vi "Eye Movement Analyser.vi"(7 "Data Output":T12) -> ()   [LabVIEW 2016] (continued)
          shift-left: dbl[][] [] -> [w1559]
          n741 = Unbundle By Name(w1562) -> ("List 1"=w1561:u16)
          n742 = Unbundle By Name(w1564) -> ("Data Channels"=w1563:dbl[][])
          n743 = Index Array(array=w1563, index (row)=w1561) -> (element=w1560:dbl[])  [unwired: 1 in]
          n744 = Build Array (concatenate)(w1559, w1560) -> (w1558:dbl[][])
        }
        n745 = Unbundle By Name(w1512) -> ("Sample Rate"=w1528:i32)
        n746 = stacked-sequence {
          tunnel: [_ w1552 _ _] -> w1514
          tunnel: [_ _ _ w1554] -> w1513
          frame #0 {
            n747 = property on="Time series Trace" class="WFGraph (strict)"("Active Cursor"=u32 0) -> ()  [unwired: 2 in, 2 out]
          }
          frame #1 {
            n748 = property on="Time series Trace" class="WFGraph (strict)"() -> ("Cursor.Cursor Position:Cursor X"=w1552:dbl)  [unwired: 2 in, 2 out]
          }
          frame #2 {
            n749 = property on="Time series Trace" class="WFGraph (strict)"("Active Cursor"=u32 1) -> ()  [unwired: 2 in, 2 out]
          }
          frame #3 {
            n750 = property on="Time series Trace" class="WFGraph (strict)"() -> ("Cursor.Cursor Position:Cursor X"=w1554:dbl)  [unwired: 2 in, 2 out]
          }
        }
        n751 = Multiply(x=w1514, y=w1528) -> (x*y=w1543:dbl)
        n752 = Multiply(x=w1513, y=w1528) -> (x*y=w1544:dbl)
        n753 = Subtract(x=w1544, y=w1543) -> (x-y=w1542:dbl)
        n754 = Decrement(x=w1542) -> (x-1=w1541:dbl)
        n755 = Array Subset(array=w1545, index (col)=w1543, length (col)=w1542) -> (w1526:dbl[][])  [unwired: 2 in]
        n756 = call-poly <vilib>:"Ramp Pattern.vi"("start"=0.0, "end"=w1541, "samples"=w1542) -> ("Ramp Pattern"=w1539:dbl[])  [unwired: 7 in, 1 out]
        n757 = for {
          tunnel: w1526 -> [w1557] mode=indexing
          tunnel: w1539 -> [w1556]
          tunnel: [w1555] -> w1527 mode=indexing
          n758 = call <vilib>:"Linear Fit.vi"("Y"=w1557, "X"=w1556) -> ("Best Linear Fit"=w1555:dbl[])  [unwired: 9 in, 4 out]
        }
        n759 = call-poly <vilib>:"Unit Vector.vi"("Input Vector"=w1518) -> ("Unit Vector"=w1511:dbl[])  [unwired: 8 in, 2 out]
        n760 = call-poly <vilib>:"Unit Vector.vi"("Input Vector"=w1517) -> ("Unit Vector"=w1510:dbl[])  [unwired: 8 in, 2 out]
        n761 = call-poly <vilib>:"Unit Vector.vi"("Input Vector"=w1516) -> ("Unit Vector"=w1508:dbl[])  [unwired: 8 in, 2 out]
        n762 = call "RotationVector_to_Quaternion-2.vi"("rotation vectors"=w1527) -> ("quaternions"=w1535:dbl[][])  [unwired: 4 in]
        n763 = Build Array (concatenate)(w1526, w1527) -> (w1504:dbl[][])
        "Fits a line to a noisy slow-phase. First 3 channels in plot window (above) must be x, y, and z eye position in that order." <- w1504
        n764 = call "Differentiate 3D.vi"("Sample Rate 4"=w1528, "Data (in)"=w1535) -> ("Data (differentiated)"=w1529:dbl[][])  [unwired: 3 in]
        n765 = call "Inverse_Quaternion-2.vi"("quaternions"=w1535) -> ("inverse quaternions"=w1530:dbl[][])  [unwired: 4 in]
        n766 = Index Array(array=w1504) -> (element #1=w1503:dbl[], element #2=w1502:dbl[], element #3=w1499:dbl[])  [unwired: 6 in]
        n767 = call "QuaternionMultiplication.vi"("quaternions B"=w1530, "quaternions A"=w1529) -> ("quaternions A x B"=w1531:dbl[][])  [unwired: 3 in]
        n768 = Divide(x=360.0, y=3.141592653589793) -> (x/y=w1534:dbl)
        n769 = Multiply(x=w1531, y=w1534) -> (x*y=w1538:dbl[][])
        n770 = call "mean_nan.vi"("Array"=w1503) -> ("Mean"=→"Mean Ch 1":dbl)  [unwired: 10 in]
        n771 = call "mean_nan.vi"("Array"=w1502) -> ("Mean"=→"Mean Ch2":dbl)  [unwired: 10 in]
        n772 = call "mean_nan.vi"("Array"=w1499) -> ("Mean"=→"Mean Ch3":dbl)  [unwired: 10 in]
        n773 = Array Subset(array=w1538, index (row)=1 ("Array Index"), length (row)=3 ("Array Index")) -> (w1525:dbl[][])  [unwired: 2 in]
        n774 = Index Array(array=w1525, index (col)=1 ("index")) -> (element=w1524:dbl[])  [unwired: 1 in]
        "X deg/s      Y deg/s      Z deg/s" <- w1524
        n775 = call-poly <vilib>:"Unit Vector.vi"("Input Vector"=w1524) -> ("Unit Vector"=w1509:dbl[])  [unwired: 8 in, 2 out]
        n776 = call-poly <vilib>:"Dot Product.vi"("Y Vector"=w1511, "X Vector"=w1509) -> ("X * Y"=w1522:dbl)  [unwired: 1 out]
        n777 = call-poly <vilib>:"Dot Product.vi"("Y Vector"=w1510, "X Vector"=w1509) -> ("X * Y"=w1523:dbl)  [unwired: 1 out]
        n778 = call-poly <vilib>:"Dot Product.vi"("Y Vector"=w1508, "X Vector"=w1509) -> ("X * Y"=w1521:dbl)  [unwired: 1 out]
        n779 = Build Array(w1522, w1523, w1521) -> (w1520:dbl[])
        n780 = Absolute Value(x=w1520) -> (abs(x)=→"HOR\n\nLARP\n\nRALP":dbl[])
      }
      frame "Mars 3D" {
        n781 = Unbundle By Name(w1568) -> ("DC file"=w1569:path)
        n782 = call "Mars3D_new.vi"("Statemachine Data IN"=w1573, "File"=w1569) -> ("stop 3"=w1572:bool, "Statemachine Data OUT"=w1570:T30)  [unwired: 8 in]
        n783 = case shown="False" w1572 {
          tunnel: [w1584 w1586] -> w1571
          tunnel: w1570 -> [w1583 w1585]
          tunnel: [w1578 w1585] -> w1565
          frame False {
            w1584 = T14[] [enum."Make Batch List", enum."Generate New Time Plot", enum."Find default parameter"] items=["--- System ---", "Panel Monitoring", "Check Save Status", "Initialize", "Initialise GUI", "Quit", "--- Import ---", "Desaccade Time Data", "Desaccade Time Data Background", "Paint Delete", "Load Batch Log File", "Make Batch List", "Update Batch List", "Delete Batch List", "Delete Temporary LVS", "Save Temporary LVS", "Check for Batch LVS", "Process 3D Chinchilla", "Find default parameter", "Mars3D old", "Chair", "EyeSeeCam", "Open last session", "Save RAW", "Auto Impulse Parameter", "Save Image", "Wireless", "Process Coils Data", "Process JHOC Data", "Process Animal Data", "Australian Data", "ASCII", "Mars 3D", "Mars 3D Training", "Position Mean Plugin", "plot generator plugin", "Human VOG system", "Optotrak", "spline", "COR", "galvanic", "Generate New Time Plot", "Make off and gains permanent", "Generate New Impulse Plot", "Defer Impulse Plot", "Fill Impulse Plot Data", "Scale Impulse Plot", "Un-Defer Impulse Plot", "Snap Impulse Cursor", "Extract Saccades", "Impulse Analyser", "NTA", "Acceleration", "Saccade Velocity", "Horizontal Align", "Vertical Align", "Delete Impulse", "Cut Before", "Cut After", "Filter Data", "Undo Last", "Redo", "Mean and STD", "Group Analyser", "Generate Report", "Phase Plots", "Gain and Phase", "Example Plugin", "Time Constant Plugin", "Export Data", "Export Time Series Data", "Append Data", "Save Data", "Load Data", "Cut in Range", "Keep in range", "Stop"] ("State stack IN")
            w1582 = 1 ("index")
            # "Use Parameter Set 0"
            n784 = Bundle By Name(cluster=w1583, "Autosort Parameter Set"=w1582) -> (w1577:T30)
            n785 = property on="Autosize Parameter Set" class="Ring (strict)"("Val(Sgnl)"=w1582) -> ()  [unwired: 2 in, 2 out]
            n786 = property on="Impulse Trace" class="WFGraph (strict)"("Value"=cluster{dbl, dbl, "Impulses":dbl[][]} {0.0, 5.0, "Impulses"=[]} ("Impulse Trace")) -> ()  [unwired: 2 in, 2 out]
            n787 = Bundle By Name(cluster=w1577, "History Length"=0, "Histpry Position"=-1, "Undo Counter"=0) -> (w1578:T30)
            n788 = property on="Tab Control" class="TabCtl (strict)"("Value"=T1."Batch Process" ("Tab Control")) -> ()  [unwired: 2 in, 2 out]
          }
          frame True {
            w1586 = T14[] [enum."Panel Monitoring"] items=["--- System ---", "Panel Monitoring", "Check Save Status", "Initialize", "Initialise GUI", "Quit", "--- Import ---", "Desaccade Time Data", "Desaccade Time Data Background", "Paint Delete", "Load Batch Log File", "Make Batch List", "Update Batch List", "Delete Batch List", "Delete Temporary LVS", "Save Temporary LVS", "Check for Batch LVS", "Process 3D Chinchilla", "Find default parameter", "Mars3D old", "Chair", "EyeSeeCam", "Open last session", "Save RAW", "Auto Impulse Parameter", "Save Image", "Wireless", "Process Coils Data", "Process JHOC Data", "Process Animal Data", "Australian Data", "ASCII", "Mars 3D", "Mars 3D Training", "Position Mean Plugin", "plot generator plugin", "Human VOG system", "Optotrak", "spline", "COR", "galvanic", "Generate New Time Plot", "Make off and gains permanent", "Generate New Impulse Plot", "Defer Impulse Plot", "Fill Impulse Plot Data", "Scale Impulse Plot", "Un-Defer Impulse Plot", "Snap Impulse Cursor", "Extract Saccades", "Impulse Analyser", "NTA", "Acceleration", "Saccade Velocity", "Horizontal Align", "Vertical Align", "Delete Impulse", "Cut Before", "Cut After", "Filter Data", "Undo Last", "Redo", "Mean and STD", "Group Analyser", "Generate Report", "Phase Plots", "Gain and Phase", "Example Plugin", "Time Constant Plugin", "Export Data", "Export Time Series Data", "Append Data", "Save Data", "Load Data", "Cut in Range", "Keep in range", "Stop"] ("State stack IN")
            # "If operation was canceld"
          }
        }
        n789 = Bundle By Name(cluster=w1568, "DC file"=path "") -> (w1567:T17)
      }
      frame "Chair" {
        n790 = Unbundle By Name(w1594) -> ("DC file"=w1589:path)
        n791 = call "Chair Plugin.vi"("DC File"=w1589, "Data IN"=w1591) -> ("Cancelled"=w1588:bool, "Data OUT"=w1590:T30)  [unwired: 8 in]
        n792 = case shown="False" w1588 {
          tunnel: [w1606 w1608] -> w1595
          tunnel: w1590 -> [w1605 w1607]
          tunnel: [w1600 w1607] -> w1587
          frame False {
            w1606 = T14[] [enum."Make Batch List", enum."Generate New Time Plot", enum."Find default parameter"] items=["--- System ---", "Panel Monitoring", "Check Save Status", "Initialize", "Initialise GUI", "Quit", "--- Import ---", "Desaccade Time Data", "Desaccade Time Data Background", "Paint Delete", "Load Batch Log File", "Make Batch List", "Update Batch List", "Delete Batch List", "Delete Temporary LVS", "Save Temporary LVS", "Check for Batch LVS", "Process 3D Chinchilla", "Find default parameter", "Mars3D old", "Chair", "EyeSeeCam", "Open last session", "Save RAW", "Auto Impulse Parameter", "Save Image", "Wireless", "Process Coils Data", "Process JHOC Data", "Process Animal Data", "Australian Data", "ASCII", "Mars 3D", "Mars 3D Training", "Position Mean Plugin", "plot generator plugin", "Human VOG system", "Optotrak", "spline", "COR", "galvanic", "Generate New Time Plot", "Make off and gains permanent", "Generate New Impulse Plot", "Defer Impulse Plot", "Fill Impulse Plot Data", "Scale Impulse Plot", "Un-Defer Impulse Plot", "Snap Impulse Cursor", "Extract Saccades", "Impulse Analyser", "NTA", "Acceleration", "Saccade Velocity", "Horizontal Align", "Vertical Align", "Delete Impulse", "Cut Before", "Cut After", "Filter Data", "Undo Last", "Redo", "Mean and STD", "Group Analyser", "Generate Report", "Phase Plots", "Gain and Phase", "Example Plugin", "Time Constant Plugin", "Export Data", "Export Time Series Data", "Append Data", "Save Data", "Load Data", "Cut in Range", "Keep in range", "Stop"] ("State stack IN")
            w1604 = 10 ("index")
            # "Use Parameter Set"
            n793 = Bundle By Name(cluster=w1605, "Autosort Parameter Set"=w1604) -> (w1599:T30)
            n794 = property on="Autosize Parameter Set" class="Ring (strict)"("Val(Sgnl)"=w1604) -> ()  [unwired: 2 in, 2 out]
            n795 = property on="Impulse Trace" class="WFGraph (strict)"("Value"=cluster{dbl, dbl, "Impulses":dbl[][]} {0.0, 5.0, "Impulses"=[]} ("Impulse Trace")) -> ()  [unwired: 2 in, 2 out]
            n796 = Bundle By Name(cluster=w1599, "History Length"=0, "Histpry Position"=-1, "Undo Counter"=0) -> (w1600:T30)
            n797 = property on="Tab Control" class="TabCtl (strict)"("Value"=T1."Batch Process" ("Tab Control")) -> ()  [unwired: 2 in, 2 out]
          }
          frame True {
            w1608 = T14[] [enum."Panel Monitoring"] items=["--- System ---", "Panel Monitoring", "Check Save Status", "Initialize", "Initialise GUI", "Quit", "--- Import ---", "Desaccade Time Data", "Desaccade Time Data Background", "Paint Delete", "Load Batch Log File", "Make Batch List", "Update Batch List", "Delete Batch List", "Delete Temporary LVS", "Save Temporary LVS", "Check for Batch LVS", "Process 3D Chinchilla", "Find default parameter", "Mars3D old", "Chair", "EyeSeeCam", "Open last session", "Save RAW", "Auto Impulse Parameter", "Save Image", "Wireless", "Process Coils Data", "Process JHOC Data", "Process Animal Data", "Australian Data", "ASCII", "Mars 3D", "Mars 3D Training", "Position Mean Plugin", "plot generator plugin", "Human VOG system", "Optotrak", "spline", "COR", "galvanic", "Generate New Time Plot", "Make off and gains permanent", "Generate New Impulse Plot", "Defer Impulse Plot", "Fill Impulse Plot Data", "Scale Impulse Plot", "Un-Defer Impulse Plot", "Snap Impulse Cursor", "Extract Saccades", "Impulse Analyser", "NTA", "Acceleration", "Saccade Velocity", "Horizontal Align", "Vertical Align", "Delete Impulse", "Cut Before", "Cut After", "Filter Data", "Undo Last", "Redo", "Mean and STD", "Group Analyser", "Generate Report", "Phase Plots", "Gain and Phase", "Example Plugin", "Time Constant Plugin", "Export Data", "Export Time Series Data", "Append Data", "Save Data", "Load Data", "Cut in Range", "Keep in range", "Stop"] ("State stack IN")
            # "If operation was canceld"
          }
        }
        n798 = Bundle By Name(cluster=w1594, "DC file"=path "") -> (w1593:T17)
      }
      frame "EyeSeeCam" {
        n799 = Unbundle By Name(w1616) -> ("DC file"=w1609:path)
        n800 = call "EyeSeeCam Plugin.vi"("DC File"=w1609, "Data IN"=w1612) -> ("Cancelled"=w1610:bool, "Data OUT"=w1611:T30)  [unwired: 8 in]
        n801 = case shown="False" w1610 {
          tunnel: [w1628 w1630] -> w1617
          tunnel: w1611 -> [w1627 w1629]
          tunnel: [w1622 w1629] -> w1613
          frame False {
            w1628 = T14[] [enum."Make Batch List", enum."Generate New Time Plot", enum."Find default parameter"] items=["--- System ---", "Panel Monitoring", "Check Save Status", "Initialize", "Initialise GUI", "Quit", "--- Import ---", "Desaccade Time Data", "Desaccade Time Data Background", "Paint Delete", "Load Batch Log File", "Make Batch List", "Update Batch List", "Delete Batch List", "Delete Temporary LVS", "Save Temporary LVS", "Check for Batch LVS", "Process 3D Chinchilla", "Find default parameter", "Mars3D old", "Chair", "EyeSeeCam", "Open last session", "Save RAW", "Auto Impulse Parameter", "Save Image", "Wireless", "Process Coils Data", "Process JHOC Data", "Process Animal Data", "Australian Data", "ASCII", "Mars 3D", "Mars 3D Training", "Position Mean Plugin", "plot generator plugin", "Human VOG system", "Optotrak", "spline", "COR", "galvanic", "Generate New Time Plot", "Make off and gains permanent", "Generate New Impulse Plot", "Defer Impulse Plot", "Fill Impulse Plot Data", "Scale Impulse Plot", "Un-Defer Impulse Plot", "Snap Impulse Cursor", "Extract Saccades", "Impulse Analyser", "NTA", "Acceleration", "Saccade Velocity", "Horizontal Align", "Vertical Align", "Delete Impulse", "Cut Before", "Cut After", "Filter Data", "Undo Last", "Redo", "Mean and STD", "Group Analyser", "Generate Report", "Phase Plots", "Gain and Phase", "Example Plugin", "Time Constant Plugin", "Export Data", "Export Time Series Data", "Append Data", "Save Data", "Load Data", "Cut in Range", "Keep in range", "Stop"] ("State stack IN")
            w1626 = 10 ("index")
            # "Use Parameter Set"
            n802 = Bundle By Name(cluster=w1627, "Autosort Parameter Set"=w1626) -> (w1621:T30)
            n803 = property on="Autosize Parameter Set" class="Ring (strict)"("Val(Sgnl)"=w1626) -> ()  [unwired: 2 in, 2 out]
            n804 = property on="Impulse Trace" class="WFGraph (strict)"("Value"=cluster{dbl, dbl, "Impulses":dbl[][]} {0.0, 5.0, "Impulses"=[]} ("Impulse Trace")) -> ()  [unwired: 2 in, 2 out]
            n805 = Bundle By Name(cluster=w1621, "History Length"=0, "Histpry Position"=-1, "Undo Counter"=0) -> (w1622:T30)
            n806 = property on="Tab Control" class="TabCtl (strict)"("Value"=T1."Batch Process" ("Tab Control")) -> ()  [unwired: 2 in, 2 out]
          }
          frame True {
            w1630 = T14[] [enum."Panel Monitoring"] items=["--- System ---", "Panel Monitoring", "Check Save Status", "Initialize", "Initialise GUI", "Quit", "--- Import ---", "Desaccade Time Data", "Desaccade Time Data Background", "Paint Delete", "Load Batch Log File", "Make Batch List", "Update Batch List", "Delete Batch List", "Delete Temporary LVS", "Save Temporary LVS", "Check for Batch LVS", "Process 3D Chinchilla", "Find default parameter", "Mars3D old", "Chair", "EyeSeeCam", "Open last session", "Save RAW", "Auto Impulse Parameter", "Save Image", "Wireless", "Process Coils Data", "Process JHOC Data", "Process Animal Data", "Australian Data", "ASCII", "Mars 3D", "Mars 3D Training", "Position Mean Plugin", "plot generator plugin", "Human VOG system", "Optotrak", "spline", "COR", "galvanic", "Generate New Time Plot", "Make off and gains permanent", "Generate New Impulse Plot", "Defer Impulse Plot", "Fill Impulse Plot Data", "Scale Impulse Plot", "Un-Defer Impulse Plot", "Snap Impulse Cursor", "Extract Saccades", "Impulse Analyser", "NTA", "Acceleration", "Saccade Velocity", "Horizontal Align", "Vertical Align", "Delete Impulse", "Cut Before", "Cut After", "Filter Data", "Undo Last", "Redo", "Mean and STD", "Group Analyser", "Generate Report", "Phase Plots", "Gain and Phase", "Example Plugin", "Time Constant Plugin", "Export Data", "Export Time Series Data", "Append Data", "Save Data", "Load Data", "Cut in Range", "Keep in range", "Stop"] ("State stack IN")
            # "If operation was canceld"
          }
        }
        n807 = Bundle By Name(cluster=w1616, "DC file"=path "") -> (w1615:T17)
      }
      frame "Mars3D old" {
        n808 = call "Mars3D_old.vi"("Statemachine Data IN"=w1636) -> ("stop 3"=w1635:bool, "Statemachine Data OUT"=w1633:T30)  [unwired: 8 in, 1 out]
        n809 = case shown="False" w1635 {
          tunnel: [w1646 w1648] -> w1634
          tunnel: w1633 -> [w1644 w1647]
          tunnel: [w1638 w1647] -> w1631
          frame False {
            w1646 = T14[] [enum."Generate New Time Plot", enum."Find default parameter"] items=["--- System ---", "Panel Monitoring", "Check Save Status", "Initialize", "Initialise GUI", "Quit", "--- Import ---", "Desaccade Time Data", "Desaccade Time Data Background", "Paint Delete", "Load Batch Log File", "Make Batch List", "Update Batch List", "Delete Batch List", "Delete Temporary LVS", "Save Temporary LVS", "Check for Batch LVS", "Process 3D Chinchilla", "Find default parameter", "Mars3D old", "Chair", "EyeSeeCam", "Open last session", "Save RAW", "Auto Impulse Parameter", "Save Image", "Wireless", "Process Coils Data", "Process JHOC Data", "Process Animal Data", "Australian Data", "ASCII", "Mars 3D", "Mars 3D Training", "Position Mean Plugin", "plot generator plugin", "Human VOG system", "Optotrak", "spline", "COR", "galvanic", "Generate New Time Plot", "Make off and gains permanent", "Generate New Impulse Plot", "Defer Impulse Plot", "Fill Impulse Plot Data", "Scale Impulse Plot", "Un-Defer Impulse Plot", "Snap Impulse Cursor", "Extract Saccades", "Impulse Analyser", "NTA", "Acceleration", "Saccade Velocity", "Horizontal Align", "Vertical Align", "Delete Impulse", "Cut Before", "Cut After", "Filter Data", "Undo Last", "Redo", "Mean and STD", "Group Analyser", "Generate Report", "Phase Plots", "Gain and Phase", "Example Plugin", "Time Constant Plugin", "Export Data", "Export Time Series Data", "Append Data", "Save Data", "Load Data", "Cut in Range", "Keep in range", "Stop"] ("State stack IN")
            w1643 = 1 ("index")
            # "Use Parameter Set 0"
            n810 = Bundle By Name(cluster=w1644, "Autosort Parameter Set"=w1643) -> (w1639:T30)
            n811 = property on="Autosize Parameter Set" class="Ring (strict)"("Val(Sgnl)"=w1643) -> ()  [unwired: 2 in, 2 out]
            n812 = local write "Tab Control"(T1."Time series Parameter" ("Tab Control")) -> ()
            n813 = Bundle By Name(cluster=w1639, "History Length"=0, "Histpry Position"=-1, "Undo Counter"=0) -> (w1638:T30)
          }
          frame True {
            w1648 = T14[] [enum."Panel Monitoring"] items=["--- System ---", "Panel Monitoring", "Check Save Status", "Initialize", "Initialise GUI", "Quit", "--- Import ---", "Desaccade Time Data", "Desaccade Time Data Background", "Paint Delete", "Load Batch Log File", "Make Batch List", "Update Batch List", "Delete Batch List", "Delete Temporary LVS", "Save Temporary LVS", "Check for Batch LVS", "Process 3D Chinchilla", "Find default parameter", "Mars3D old", "Chair", "EyeSeeCam", "Open last session", "Save RAW", "Auto Impulse Parameter", "Save Image", "Wireless", "Process Coils Data", "Process JHOC Data", "Process Animal Data", "Australian Data", "ASCII", "Mars 3D", "Mars 3D Training", "Position Mean Plugin", "plot generator plugin", "Human VOG system", "Optotrak", "spline", "COR", "galvanic", "Generate New Time Plot", "Make off and gains permanent", "Generate New Impulse Plot", "Defer Impulse Plot", "Fill Impulse Plot Data", "Scale Impulse Plot", "Un-Defer Impulse Plot", "Snap Impulse Cursor", "Extract Saccades", "Impulse Analyser", "NTA", "Acceleration", "Saccade Velocity", "Horizontal Align", "Vertical Align", "Delete Impulse", "Cut Before", "Cut After", "Filter Data", "Undo Last", "Redo", "Mean and STD", "Group Analyser", "Generate Report", "Phase Plots", "Gain and Phase", "Example Plugin", "Time Constant Plugin", "Export Data", "Export Time Series Data", "Append Data", "Save Data", "Load Data", "Cut in Range", "Keep in range", "Stop"] ("State stack IN")
            # "If operation was canceld"
          }
        }
      }
      frame "Process 3D Chinchilla" {
        n814 = call "Mars3D_new.vi"("Statemachine Data IN"=w1651) -> ("Statemachine Data OUT"=w1652:T30)  [unwired: 9 in, 1 out]
        n815 = case shown="False" FALSE {
          tunnel: [w1660 w1662] -> w1654
          tunnel: w1652 -> [w1658 w1661]
          tunnel: [w1657 w1661] -> w1649
          frame False {
            w1660 = T14[] [enum."Generate New Time Plot"] items=["--- System ---", "Panel Monitoring", "Check Save Status", "Initialize", "Initialise GUI", "Quit", "--- Import ---", "Desaccade Time Data", "Desaccade Time Data Background", "Paint Delete", "Load Batch Log File", "Make Batch List", "Update Batch List", "Delete Batch List", "Delete Temporary LVS", "Save Temporary LVS", "Check for Batch LVS", "Process 3D Chinchilla", "Find default parameter", "Mars3D old", "Chair", "EyeSeeCam", "Open last session", "Save RAW", "Auto Impulse Parameter", "Save Image", "Wireless", "Process Coils Data", "Process JHOC Data", "Process Animal Data", "Australian Data", "ASCII", "Mars 3D", "Mars 3D Training", "Position Mean Plugin", "plot generator plugin", "Human VOG system", "Optotrak", "spline", "COR", "galvanic", "Generate New Time Plot", "Make off and gains permanent", "Generate New Impulse Plot", "Defer Impulse Plot", "Fill Impulse Plot Data", "Scale Impulse Plot", "Un-Defer Impulse Plot", "Snap Impulse Cursor", "Extract Saccades", "Impulse Analyser", "NTA", "Acceleration", "Saccade Velocity", "Horizontal Align", "Vertical Align", "Delete Impulse", "Cut Before", "Cut After", "Filter Data", "Undo Last", "Redo", "Mean and STD", "Group Analyser", "Generate Report", "Phase Plots", "Gain and Phase", "Example Plugin", "Time Constant Plugin", "Export Data", "Export Time Series Data", "Append Data", "Save Data", "Load Data", "Cut in Range", "Keep in range", "Stop"] ("State stack IN")
            w1656 = 3 ("index")
            # "Use Parameter Set 0"
            n816 = Bundle By Name(cluster=w1658, "Autosort Parameter Set"=w1656) -> (w1657:T30)
            n817 = property on="Autosize Parameter Set" class="Ring (strict)"("Val(Sgnl)"=w1656) -> ()  [unwired: 2 in, 2 out]
            n818 = local write "Tab Control"(T1."Time series Parameter" ("Tab Control")) -> ()
          }
          frame True {
            w1662 = T14[] [enum."Panel Monitoring"] items=["--- System ---", "Panel Monitoring", "Check Save Status", "Initialize", "Initialise GUI", "Quit", "--- Import ---", "Desaccade Time Data", "Desaccade Time Data Background", "Paint Delete", "Load Batch Log File", "Make Batch List", "Update Batch List", "Delete Batch List", "Delete Temporary LVS", "Save Temporary LVS", "Check for Batch LVS", "Process 3D Chinchilla", "Find default parameter", "Mars3D old", "Chair", "EyeSeeCam", "Open last session", "Save RAW", "Auto Impulse Parameter", "Save Image", "Wireless", "Process Coils Data", "Process JHOC Data", "Process Animal Data", "Australian Data", "ASCII", "Mars 3D", "Mars 3D Training", "Position Mean Plugin", "plot generator plugin", "Human VOG system", "Optotrak", "spline", "COR", "galvanic", "Generate New Time Plot", "Make off and gains permanent", "Generate New Impulse Plot", "Defer Impulse Plot", "Fill Impulse Plot Data", "Scale Impulse Plot", "Un-Defer Impulse Plot", "Snap Impulse Cursor", "Extract Saccades", "Impulse Analyser", "NTA", "Acceleration", "Saccade Velocity", "Horizontal Align", "Vertical Align", "Delete Impulse", "Cut Before", "Cut After", "Filter Data", "Undo Last", "Redo", "Mean and STD", "Group Analyser", "Generate Report", "Phase Plots", "Gain and Phase", "Example Plugin", "Time Constant Plugin", "Export Data", "Export Time Series Data", "Append Data", "Save Data", "Load Data", "Cut in Range", "Keep in range", "Stop"] ("State stack IN")
            # "If operation was canceld"
          }
        }
      }
      frame "Wireless" {
        n819 = File Dialog() -> (0:w1678:errorcluster, 3:w1664:path)  [unwired: 7 in, 2 out]
        n820 = Unbundle(w1678) -> ()  [unwired: 3 out]
        n821 = call <vilib>:"Read Lines From File.vi"("file path (dialog if empty)"=w1664, "number of lines (all:-1)"=16) -> ("line string"=w1677:string, "mark after read (chars.)"=w1673:i32)  [unwired: 4 in, 2 out]
        n822 = call-poly <vilib>:"Read From Spreadsheet File.vi"("start of read offset (chars.:0)"=w1673, "file path (dialog if empty)"=w1664) -> ("all rows"=w1668:dbl[][])  [unwired: 5 in, 4 out]
        n823 = Scan From String(input string=w1677) -> (remaining string=w1675:string, output 1=w1676:dbl)  [unwired: 4 in, 2 out]
        n824 = To Long Integer(number=w1676) -> (32bit integer=w1669:i32)
        n825 = call <vilib>:"Trim Whitespace.vi"("string"=w1675) -> ("trimmed string"=w1674:string)  [unwired: 1 in]
        n826 = while {
          shift-right: [w1684] -> _
          shift-left: w1674 -> [w1685]
          tunnel: [w1683] -> w1667 mode=indexing
          stop <- w1681 continue-if-true
          n827 = Match Pattern(string=w1685, regular expression="\t") -> (before substring=w1683:string, after substring=w1684:string, offset past match=w1680:i32)  [unwired: 1 in, 1 out]
          n828 = Increment(x=w1680) -> (x+1=w1682:i32)
          n829 = Not Equal To 0?(x=w1682) -> (x != 0?=w1681:bool)
        }
        n830 = Bundle By Name(cluster=w1666, "Data File.Data Channels"=w1668, "Data File.Sample Rate"=w1669, "Data File.Channel List"=w1667) -> (w1665:T30)
      }
      frame "Mars 3D Training" {
        w1691 = T14[] [enum."Generate New Time Plot"] items=["--- System ---", "Panel Monitoring", "Check Save Status", "Initialize", "Initialise GUI", "Quit", "--- Import ---", "Desaccade Time Data", "Desaccade Time Data Background", "Paint Delete", "Load Batch Log File", "Make Batch List", "Update Batch List", "Delete Batch List", "Delete Temporary LVS", "Save Temporary LVS", "Check for Batch LVS", "Process 3D Chinchilla", "Find default parameter", "Mars3D old", "Chair", "EyeSeeCam", "Open last session", "Save RAW", "Auto Impulse Parameter", "Save Image", "Wireless", "Process Coils Data", "Process JHOC Data", "Process Animal Data", "Australian Data", "ASCII", "Mars 3D", "Mars 3D Training", "Position Mean Plugin", "plot generator plugin", "Human VOG system", "Optotrak", "spline", "COR", "galvanic", "Generate New Time Plot", "Make off and gains permanent", "Generate New Impulse Plot", "Defer Impulse Plot", "Fill Impulse Plot Data", "Scale Impulse Plot", "Un-Defer Impulse Plot", "Snap Impulse Cursor", "Extract Saccades", "Impulse Analyser", "NTA", "Acceleration", "Saccade Velocity", "Horizontal Align", "Vertical Align", "Delete Impulse", "Cut Before", "Cut After", "Filter Data", "Undo Last", "Redo", "Mean and STD", "Group Analyser", "Generate Report", "Phase Plots", "Gain and Phase", "Example Plugin", "Time Constant Plugin", "Export Data", "Export Time Series Data", "Append Data", "Save Data", "Load Data", "Cut in Range", "Keep in range", "Stop"] ("State stack IN")
        w1692 = 5 ("Autosort Parameter Set")
        n831 = Unbundle By Name(w1696) -> ("Experiment data path"=w1697:path)
        n832 = File Dialog(11:w1697) -> (3:w1702:path)  [unwired: 6 in, 3 out]
        n833 = disable-structure shown="Enabled" {
          disable-tunnel: [string[] ["Time", "Motor-Pos", "Motor-Vel", "Horizontal-Pos", "Horizontal-Vel", "Vertical-Pos", "Vertical-Vel", "Trigger"] ("Data File.Channel List") string[] ["Motor", "Projector", "Projector Error"] ("Data File.Channel List")] -> w1701
          frame Disabled {
          }
          frame Enabled {
          }
        }
        n834 = call <vilib>:"Read Lines From File.vi"("file path (dialog if empty)"=w1702, "number of lines (all:-1)"=17) -> ("new file path (Not A Path if cancelled)"=w1694:path, "mark after read (chars.)"=w1706:i32)  [unwired: 4 in, 2 out]
        n835 = call-poly <vilib>:"Read From Spreadsheet File.vi"("start of read offset (chars.:0)"=w1706, "file path (dialog if empty)"=w1702) -> ("all rows"=w1699:dbl[][])  [unwired: 5 in, 4 out]
        n836 = Strip Path(path=w1694) -> (stripped path=w1693:path)  [unwired: 1 out]
        n837 = Bundle By Name(cluster=w1696, "Experiment data path"=w1693) -> (w1695:T30)
        n838 = Transpose 2D Array(2D array=w1699) -> (transposed array=w1698:dbl[][])
        n839 = property on="Autosize Parameter Set" class="Ring (strict)"("Val(Sgnl)"=w1692) -> ()  [unwired: 2 in, 2 out]
        n840 = Bundle By Name(cluster=w1695, "Data File.Data Channels"=w1698, "Data File.Sample Rate"=1000, "Data File.Channel List"=w1701, "Autosort Parameter Set"=w1692, "Parameter Time Series"=T2 [], "Parameter Impuls Series"=T8 [{"Color"=4652800, "Visible"=TRUE, "Channel"=0, "Invert"=FALSE, "Desaccade"=FALSE, "Offset"=0.0, "Gain"=1.0}, {"Color"=16860, "Visible"=TRUE, "Channel"=1, "Invert"=FALSE, "Desaccade"=FALSE, "Offset"=0.0, "Gain"=1.0}]) -> (w1703:T30)
        n841 = local write "Tab Control"(T1."Time series Parameter" ("Tab Control")) -> ()
      }
      frame "Human VOG system" {
        n842 = call "Human VOG.vi"() -> ("Data Output"=w1710:T12)  [unwired: 15 in]
        n843 = Bundle By Name(cluster=w1712, "Data File"=w1710) -> (w1711:T30)
      }
      frame "Impulse Analyser" {
        n844 = Unbundle By Name(w1720) -> ("Data File"=w1724:T12)
        n845 = Unbundle By Name(w1724) -> ("Sample Rate"=w1736:i32)
        n846 = Unbundle By Name(w1724) -> ("Data Channels"=w1746:dbl[][])
        n847 = call "Find A Channel.vi"("element"="Hx Velocity-in-Head", "Data Output"=w1724) -> ("Signal (V)"=w1751:dbl[])
        n848 = call "Find A Channel.vi"("element"="Hy Velocity-in-Head", "Data Output"=w1724) -> ("Signal (V)"=w1750:dbl[])
        n849 = call "Find A Channel.vi"("element"="Hz Velocity-in-Head", "Data Output"=w1724) -> ("Signal (V)"=w1749:dbl[])
        n850 = call "Find A Channel.vi"("element"="Hl Velocity-in-Head", "Data Output"=w1724) -> ("Signal (V)"=w1748:dbl[])
        n851 = call "Find A Channel.vi"("element"="Hr Velocity-in-Head", "Data Output"=w1724) -> ("Signal (V)"=w1747:dbl[])
        n852 = Index Array(array=w1746, index (row)="Trigger Channel (Other)") -> (element=w1745:dbl[])  [unwired: 1 in]
        n853 = local read "Interpolate"() -> (w1733:bool)
        n854 = Build Array(w1751, w1750, w1749, w1748, w1747, w1745) -> (w1735:dbl[][])
        n855 = local read "Other Trigger channel"() -> (w1723:bool)
        n856 = local read "Cross Correlation"() -> (w1732:bool)
        n857 = case shown="False" w1733 {
          tunnel: w1735 -> [w1756 w1759]
          tunnel: [w1756 w1758] -> w1734
          frame False {
          }
          frame True {
            n858 = call "interp type 2.vi"("NaN"=w1759, "Remove front and end"=TRUE) -> ("Interpolated"=w1758:dbl[][])
          }
        }
        n859 = local read "Accel Threshold [TH-1]"() -> (w1729:dbl)
        n860 = Unbundle By Name(w1720) -> ("Data File.Sample Rate"=w1726:i32)
        n861 = local read "Tolerance [ms]"() -> (w1730:dbl)
        n862 = local read "Impulse Plane 2"() -> (w1728:T9)
        n863 = local read "Impulse dir"() -> (w1727:bool)
        n864 = call "Impulse_Correlation.vi"("Head Velocity"=w1734, "Trigger"="Trigger Method", "Cross-Correlation"=w1732, "Impulse surround"="Impulse surround", "First Pass Criterea"="Impulse Characteristics", "Sample Rate"=w1736, "Other Trigger"=w1723) -> ("Impulse Array"=w1721:T11)  [unwired: 8 in]
        n865 = Bundle("Tolerance [ms]"=w1730, "Accel Threshold [TH-1]"=w1729, "Sample Rate"=w1726, "Impulse Plane 2"=w1728, "Impulse dir"=w1727) -> (w1725:T32)  [unwired: 1 in]
        n866 = case shown="True" w1723 {
          frame False {
            n867 = property on="Impulse Plane 2" class="Enum (strict)"("Val(Sgnl)"=T9."Yaw" ("Impulse Plane")) -> ()  [unwired: 2 in, 2 out]
          }
          frame True {
            n868 = property on="Impulse Plane 2" class="Enum (strict)"("Val(Sgnl)"=T9."Other" ("Impulse Plane")) -> ()  [unwired: 2 in, 2 out]
          }
        }
        n869 = local write "Impulse Positions"(w1721) -> ()
        n870 = call "Add History.vi"("Data IN"=w1720, "Impulse Positions"=w1721) -> ("Data OUT"=w1719:T30)  [unwired: 9 in]
        n871 = Bundle By Name(cluster=w1719, "Impulse Positions"=w1721, "desaccading parameters"=w1725) -> (w1752:T30)
      }
      frame "Generate New Impulse Plot" {
        w1760 = T14[] [enum."Defer Impulse Plot", enum."Fill Impulse Plot Data", enum."Scale Impulse Plot", enum."Un-Defer Impulse Plot"] items=["--- System ---", "Panel Monitoring", "Check Save Status", "Initialize", "Initialise GUI", "Quit", "--- Import ---", "Desaccade Time Data", "Desaccade Time Data Background", "Paint Delete", "Load Batch Log File", "Make Batch List", "Update Batch List", "Delete Batch List", "Delete Temporary LVS", "Save Temporary LVS", "Check for Batch LVS", "Process 3D Chinchilla", "Find default parameter", "Mars3D old", "Chair", "EyeSeeCam", "Open last session", "Save RAW", "Auto Impulse Parameter", "Save Image", "Wireless", "Process Coils Data", "Process JHOC Data", "Process Animal Data", "Australian Data", "ASCII", "Mars 3D", "Mars 3D Training", "Position Mean Plugin", "plot generator plugin", "Human VOG system", "Optotrak", "spline", "COR", "galvanic", "Generate New Time Plot", "Make off and gains permanent", "Generate New Impulse Plot", "Defer Impulse Plot", "Fill Impulse Plot Data", "Scale Impulse Plot", "Un-Defer Impulse Plot", "Snap Impulse Cursor", "Extract Saccades", "Impulse Analyser", "NTA", "Acceleration", "Saccade Velocity", "Horizontal Align", "Vertical Align", "Delete Impulse", "Cut Before", "Cut After", "Filter Data", "Undo Last", "Redo", "Mean and STD", "Group Analyser", "Generate Report", "Phase Plots", "Gain and Phase", "Example Plugin", "Time Constant Plugin", "Export Data", "Export Time Series Data", "Append Data", "Save Data", "Load Data", "Cut in Range", "Keep in range", "Stop"] ("array")
        n872 = Build Array (concatenate)(w1762, w1760) -> (w1761:T14[])
        n873 = Bundle By Name(cluster=w1767, "Session saved?"=FALSE) -> (w1766:T17)
      }
      frame "Defer Impulse Plot" {
        n874 = control-ref of="Impulse Trace"() -> (w1773:refnum<vi>)
        n875 = call "Constructor.vi"("Graph Reference"=w1773) -> ("Graph Manager out"=w1772:refnum<class "Graph Manager.lvclass">)  [unwired: 10 in]
        n876 = call-dynamic "Defer Panel Updates.vi"("Defer Panel Updates"=TRUE, "Graph Manager in"=w1772) -> ()  [unwired: 8 in, 2 out]
      }
      frame "Fill Impulse Plot Data" {
        # "Setup Graph Object with the correct sample rate"
        # "Get Impulses to draw from internal data"
        n877 = local read "Spline balance parameter"() -> (w1790:dbl)
        n878 = Unbundle By Name(w1785) -> ("Data File"=w1797:T12, "Impulse Positions"=w1796:T11, "Parameter Impuls Series"=w1782:T8, "desacc"=w1795:T31)
        n879 = Unbundle By Name(w1785) -> ("Data File.Sample Rate"=w1788:i32)
        n880 = local read "Capture Saccade"() -> (w1793:bool)
        n881 = local read "Display Saccade"() -> (w1789:bool)
        n882 = local read "Impulse Plane 2"() -> (w1792:T9)
        n883 = control-ref of="Impulse Trace"() -> (w1799:refnum<vi>)
        n884 = local read "Impulse dir"() -> (w1794:bool)
        n885 = local read "Interpolate"() -> (w1791:bool)
        n886 = call "Constructor.vi"("Graph Reference"=w1799) -> ("Graph Manager out"=w1798:refnum<class "Graph Manager.lvclass">)  [unwired: 10 in]
        n887 = call "Couple Head Impulse Traces.vi"("Data Input"=w1797, "Impulse Positions"=w1796, "Impulse Direction +ve?"=w1794, "Capture Saccade"=w1793, "Impulse Plane"=w1792, "Plot Selection 2"=w1782, "desacc"=w1795, "Interpolate"=w1791, "Display Saccade"=w1789, "balance parameter (s-pline Parameter)"=w1790) -> ("Impulse Positions 2"=w1787:T11, "No Impulses"=w1783:i32, "Impulses"=w1784:dbl[][])  [unwired: 6 in, 1 out]
        n888 = call-dynamic "Set Sample Rate.vi"("Sample Rate"=w1788, "Graph Manager in"=w1798) -> ("error out"=w1780:errorcluster, "Graph Manager out"=w1781:refnum<class "Graph Manager.lvclass">)  [unwired: 8 in]
        n889 = Bundle By Name(cluster=w1785, "Impulse Positions"=w1787, "No. Imp"=w1783) -> (w1786:T30)
        n890 = for {
          tunnel: w1782 -> [w1836] mode=indexing
          shift-right: [w1840] -> _
          shift-left: w1784 -> [w1841]
          tunnel: w1783 -> [w1839]
          shift-right: [w1827] -> w1778
          shift-left: w1781 -> [w1842]
          shift-right: [w1826] -> w1777
          shift-left: w1780 -> [w1843]
          # "Add the impulse data to the graph"
          # "Puts plots in the order expected by paint delete."
          # "Visibility"
          # "Colour"
          # "Add Data"
          # "Get the channel's impulse data"
          # "For each channel..."
          n891 = Unbundle By Name(w1836) -> ("Visible"=w1825:bool, "Color"=w1834:u32, "Invert"=w1835:bool)
          n892 = Delete From Array(array=w1841, length=w1839, index (row)=0) -> (deleted portion=w1838:dbl[][], array with subset deleted=w1840:dbl[][])  [unwired: 1 in]
          n893 = call-dynamic "Add Channel Data.vi"("Inverted?"=w1835, "error in (no error)"=w1843, "Layer"=enum16{"Top", "Bottom"}."Bottom", "Channel Data"=w1838, "Graph Manager in"=w1842) -> ("error out"=w1833:errorcluster, "Channel ID"=w1831:i32, "Graph Manager out"=w1832:refnum<class "Graph Manager.lvclass">)  [unwired: 4 in]
          n894 = call-dynamic "Set Colour.vi"("error in (no error)"=w1833, "Color Box"=w1834, "Channel in"=w1831, "Graph Manager in"=w1832) -> ("error out"=w1829:errorcluster, "Channel out"=w1828:i32, "Graph Manager out"=w1830:refnum<class "Graph Manager.lvclass">)  [unwired: 5 in]
          n895 = call-dynamic "Set Visibility.vi"("error in (no error)"=w1829, "Visible? (F)"=w1825, "Channel in"=w1828, "Graph Manager in"=w1830) -> ("error out"=w1826:errorcluster, "Graph Manager out"=w1827:refnum<class "Graph Manager.lvclass">)  [unwired: 5 in, 1 out]
        }
        n896 = local read "Mean and STD"() -> (w1779:bool)
        n897 = case shown="False" w1779 {
          tunnel: w1778 -> [w1805 w1819]
          tunnel: w1777 -> [w1804 w1818]
          frame False {
            # "Highlight selected trace."
            # "Draw all data on the graph"
            # "Show individual traces on the graph."
            n898 = call-dynamic "Draw Normal.vi"("Auto Defer Panel Updates? (T)"=FALSE, "error in (no error)"=w1804, "Graph Manager in"=w1805) -> ("error out"=w1806:errorcluster, "Graph Manager out"=w1807:refnum<class "Graph Manager.lvclass">)  [unwired: 7 in]
            n899 = local read "Trace"() -> (w1810:i32)
            n900 = Greater Or Equal To 0?(x=w1810) -> (x >= 0?=w1809:bool)
            n901 = case shown="True" w1809 {
              tunnel: w1807 -> [w1812 w1817]
              tunnel: w1806 -> [w1811 w1816]
              tunnel: w1810 -> [_ w1815]
              tunnel: [w1812 w1814] -> _
              tunnel: [w1811 w1813] -> _
              frame False {
              }
              frame True {
                n902 = call "Highlight Trace.vi"("error in (no error)"=w1816, "Trace"=w1815, "Graph Manager in"=w1817) -> ("error out"=w1813:errorcluster, "Graph Manager out"=w1814:refnum<class "Graph Manager.lvclass">)  [unwired: 7 in]
              }
            }
          }
          frame True {
            # "Draw Mean. Deferred updates handled elsewhere..."
            # "Set Mean"
            # "Show mean traces on the graph."
            n903 = call-dynamic "Set all channels Mean.vi"("error in (no error)"=w1818, "Boolean"=TRUE, "Graph Manager in"=w1819) -> ("error out"=w1822:errorcluster, "Graph Manager out"=w1823:refnum<class "Graph Manager.lvclass">)  [unwired: 7 in]
            n904 = call-dynamic "Draw Mean.vi"("Auto Defer Panel Updates? (T)"=FALSE, "error in (no error)"=w1822, "Graph Manager in"=w1823) -> ()  [unwired: 7 in, 2 out]
          }
        }
      }
      frame "Scale Impulse Plot" {
        n905 = control-ref of="Impulse Trace"() -> (w1851:refnum<vi>)
        n906 = call "Constructor.vi"("Graph Reference"=w1851) -> ("Graph Manager out"=w1850:refnum<class "Graph Manager.lvclass">)  [unwired: 10 in]
        n907 = local read "Fixed Time"() -> (w1847:bool)
        n908 = case shown="False" w1847 {
          tunnel: w1850 -> [w1861 w1862]
          tunnel: [w1860 w1862] -> w1849
          tunnel: [w1859 _] -> w1848
          frame False {
            n909 = call "Auto Scale.vi"("Scale (X AND Y)"=enum16{"X AND Y", "X", "Y", "NONE"}."X", "Graph Manager in"=w1861) -> ("error out"=w1859:errorcluster, "Graph Manager out"=w1860:refnum<class "Graph Manager.lvclass">)  [unwired: 8 in]
          }
          frame True {
          }
        }
        n910 = local read "Fixed Amplitude"() -> (w1846:bool)
        n911 = case shown="False" w1846 {
          tunnel: w1849 -> [w1857 _]
          tunnel: w1848 -> [w1856 _]
          frame False {
            n912 = call "Auto Scale.vi"("error in (no error)"=w1856, "Scale (X AND Y)"=enum16{"X AND Y", "X", "Y", "NONE"}."Y", "Graph Manager in"=w1857) -> ()  [unwired: 7 in, 2 out]
          }
          frame True {
          }
        }
      }
      frame "Un-Defer Impulse Plot" {
        n913 = control-ref of="Impulse Trace"() -> (w1865:refnum<vi>)
        n914 = call "Constructor.vi"("Graph Reference"=w1865) -> ("Graph Manager out"=w1864:refnum<class "Graph Manager.lvclass">)  [unwired: 10 in]
        n915 = call-dynamic "Defer Panel Updates.vi"("Defer Panel Updates"=FALSE, "Graph Manager in"=w1864) -> ()  [unwired: 8 in, 2 out]
      }
      frame "Snap Impulse Cursor" {
        n916 = property on="Impulse Trace" class="WFGraph (strict)"() -> ("Cursor.CursorMode"=w1873:u32)  [unwired: 2 in, 2 out]
        n917 = Unbundle By Name(w1872) -> ("No. Imp"=w1871:i32)
        n918 = case shown="Default" w1873 {
          tunnel: w1871 -> [_ w1879]
          frame 0 {
            # "Cursor is in free mode. No snapping required."
          }
          frame Default {
            # "Snap to the closest plot."
            # "Enables Dragging to other plots."
            # "Shortest Y distance to the cursor."
            # "Cursor is in a snapping mode. Go ahead and snap it."
            n919 = property on="Impulse Trace" class="WFGraph (strict)"() -> ("Value"=w1891:cluster{dbl, dbl, "Impulses":dbl[][]})  [unwired: 2 in, 2 out]
            n920 = property on="Impulse Trace" class="WFGraph (strict)"() -> ("Cursor.Cursor Y"=w1886:dbl, "Cursor.Cursor X"=w1887:dbl)  [unwired: 2 in, 2 out]
            n921 = Unbundle(w1891) -> (w1890:dbl, "Impulses"=w1889:dbl[][])  [unwired: 1 out]
            n922 = Divide(x=w1887, y=w1890) -> (x/y=w1888:dbl)
            n923 = for {
              tunnel: w1889 -> [w1900] mode=indexing
              tunnel: w1888 -> [w1899]
              tunnel: w1886 -> [w1898]
              shift-right: [w1894] -> _
              shift-left: inf -> [w1895]
              tunnel: [w1893] -> w1880 if=w1892
              i -> [w1893]
              # "Keep this plot # if it is the closest to the cursor so far."
              n924 = property on="Impulse Trace" class="WFGraph (strict)"("Active Plot"=w1893) -> ("Plot.Visible?"=w1897:bool)  [unwired: 2 in, 2 out]
              n925 = case shown="True" w1897 {
                tunnel: w1900 -> [_ w1907]
                tunnel: w1899 -> [_ w1906]
                tunnel: w1898 -> [_ w1905]
                tunnel: [inf w1902] -> w1896
                frame False {
                  # "Plot isn't visible. It is not a candidate for snapping to."
                }
                frame True {
                  # "Plot is visible. Check it's Y distance to the cursor."
                  n926 = Interpolate 1D Array(1:w1906, 2:w1907) -> (0:w1904:dbl)
                  n927 = Subtract(x=w1905, y=w1904) -> (x-y=w1903:dbl)
                  n928 = Absolute Value(x=w1903) -> (abs(x)=w1902:dbl)
                }
              }
              n929 = Less?(x=w1896, y=w1895) -> (x < y?=w1892:bool)
              n930 = Select(t=w1896, s=w1892, f=w1895) -> (s? t:f=w1894:dbl)
            }
            n931 = Quotient & Remainder(x=w1880, y=w1879) -> (x-y*floor(x/y)=w1878:i32)  [unwired: 1 out]
            n932 = property on="Impulse Trace" class="WFGraph (strict)"("Cursor.Cursor Plot"=w1880, "Cursor.Cursor Plot"=-1) -> (error out=w1883:errorcluster)  [unwired: 2 in, 1 out]
            n933 = local write "Trace"(w1878) -> ()
            n934 = property on="Impulse Trace" class="WFGraph (strict)"(error in=w1883) -> ("Cursor.Cursor X"=w1882:dbl, "Cursor.Cursor Y"=w1881:dbl)  [unwired: 1 in, 2 out]
            n935 = property on="Impuls Cursor X" class="DigNum (strict)"("Value"=w1882) -> ()  [unwired: 2 in, 2 out]
            n936 = property on="Impuls Cursor Y" class="DigNum (strict)"("Value"=w1881) -> ()  [unwired: 2 in, 2 out]
          }
        }
      }
      frame "Extract Saccades" {
        n937 = disable-structure shown="Enabled" {
          disable-tunnel: w1912 -> [w1914 w1917]
          disable-tunnel: [_ w1916] -> w1908
          frame Disabled {
            n938 = call "Saccade-Analyser.vi"("EMA-Data IN"=w1914) -> ()  [unwired: 3 in]
          }
          frame Enabled {
            n939 = call "SaccadeAnalyser - Main.vi"("Data IN"=w1917) -> ("error out"=w1915:errorcluster, "Data OUT"=w1916:T30)  [unwired: 9 in]
            n940 = call <vilib>:"Simple Error Handler.vi"("error in (no error)"=w1915) -> ()  [unwired: 4 in, 5 out]
          }
        }
      }
      frame "Mean and STD" {
        n941 = disable-structure shown="Enabled" {
          disable-tunnel: w1920 -> [w1925 _]
          frame Disabled {
            w1929 = TRUE ("Mean and STD")
            n942 = Unbundle By Name(w1925) -> ("Impulse Positions"=w1936:T11, "desacc"=w1923:T31)
            n943 = local read "Parameter Impuls Series"() -> (w1933:T8)
            n944 = Unbundle By Name(w1925) -> ("Data File"=w1924:T12)
            n945 = Unbundle By Name(w1924) -> ("Sample Rate"=w1926:i32)
            n946 = local read "Impulse Plane 2"() -> (w1934:T9)
            n947 = local read "Impulse dir"() -> (w1935:bool)
            n948 = local read "Spline balance parameter"() -> (w1927:dbl)
            n949 = call "Couple Head Impulse Traces.vi"("Data Input"=w1924, "Impulse Positions"=w1936, "Impulse Direction +ve?"=w1935, "Impulse Plane"=w1934, "Mean and STD"=w1929, "Plot Selection 2"=w1933, "Export"=FALSE, "desacc"=w1923, "Interpolate"=w1929, "S-pline"="S-pline", "balance parameter (s-pline Parameter)"=w1927) -> ("Mean and STD"=w1931:dbl[][])  [unwired: 5 in, 3 out]
            n950 = To Double Precision Float(number=w1926) -> (double precision float=w1932:dbl)
            n951 = stacked-sequence {
              tunnel: w1931 -> [w1940 _ _]
              tunnel: w1933 -> [_ _ w2035]
              tunnel: w1932 -> [w1937 _ _]
              frame #0 {
                n952 = Divide(x=1000.0 ("y"), y=w1937) -> (x/y=w1943:dbl)
                n953 = case shown="True" "Change coord" {
                  tunnel: w1940 -> [w1945 w1998]
                  tunnel: [w1945 w1962] -> w1938
                  frame False {
                  }
                  frame True {
                    n954 = Index Array(array=w1998, index (row)=0) -> (element=w1997:dbl[])  [unwired: 1 in]
                    n955 = Index Array(array=w1998, index (row)=3) -> (element=w1996:dbl[])  [unwired: 1 in]
                    n956 = Index Array(array=w1998, index (row)=6) -> (element=w1995:dbl[])  [unwired: 1 in]
                    n957 = Index Array(array=w1998, index (row)=1) -> (element=w1994:dbl[])  [unwired: 1 in]
                    n958 = Index Array(array=w1998, index (row)=4) -> (element=w1993:dbl[])  [unwired: 1 in]
                    n959 = Index Array(array=w1998, index (row)=7) -> (element=w1992:dbl[])  [unwired: 1 in]
                    n960 = Index Array(array=w1998, index (row)=2) -> (element=w1991:dbl[])  [unwired: 1 in]
                    n961 = Index Array(array=w1998, index (row)=5) -> (element=w1990:dbl[])  [unwired: 1 in]
                    n962 = Index Array(array=w1998, index (row)=8) -> (element=w1989:dbl[])  [unwired: 1 in]
                    n963 = call "Fick to Rotation Matrix.vi"("T"="T", "V"="V", "H"="H") -> ("Rotation Matrix"=w1988:dbl[][])
                    n964 = for {
                      tunnel: w1997 -> [w2025] mode=indexing
                      tunnel: w1996 -> [w2024] mode=indexing
                      tunnel: w1995 -> [w2023] mode=indexing
                      tunnel: w1994 -> [w2021] mode=indexing
                      tunnel: w1993 -> [w2019] mode=indexing
                      tunnel: w1992 -> [w2018] mode=indexing
                      tunnel: w1991 -> [w2020] mode=indexing
                      tunnel: w1990 -> [w2017] mode=indexing
                      tunnel: w1989 -> [w2016] mode=indexing
                      tunnel: w1988 -> [w2014]
                      tunnel: [w2008] -> w1975 mode=indexing
                      n965 = Build Array(w2025, w2024, w2023) -> (w2022:dbl[])
                      n966 = Build Array(w2021, w2019, w2018) -> (w2015:dbl[])
                      n967 = Build Array(w2020, w2017, w2016) -> (w2013:dbl[])
                      n968 = call-poly <vilib>:"A x B.vi"("Vector"=w2022, "A"=w2014) -> ("A x Vector"=w2012:dbl[])  [unwired: 1 out]
                      n969 = call-poly <vilib>:"A x B.vi"("Vector"=w2015, "A"=w2014) -> ("A x Vector"=w2011:dbl[])  [unwired: 1 out]
                      n970 = call-poly <vilib>:"A x B.vi"("Vector"=w2013, "A"=w2014) -> ("A x Vector"=w2010:dbl[])  [unwired: 1 out]
                      n971 = for {
                        tunnel: w2012 -> [w2030] mode=indexing
                        tunnel: w2011 -> [w2029] mode=indexing
                        tunnel: w2010 -> [w2028] mode=indexing
                        shift-right: [w2027] -> w2008
                        shift-left: dbl[] [] -> [w2026]
                        n972 = Build Array (concatenate)(w2026, w2030, w2029, w2028) -> (w2027:dbl[])
                      }
                    }
                    n973 = Transpose 2D Array(2D array=w1975) -> (transposed array=w1961:dbl[][])
                    n974 = Index Array(array=w1961, index (row)=0) -> (element=w1974:dbl[])  [unwired: 1 in]
                    n975 = Index Array(array=w1961, index (row)=3) -> (element=w1973:dbl[])  [unwired: 1 in]
                    n976 = Index Array(array=w1961, index (row)=6) -> (element=w1972:dbl[])  [unwired: 1 in]
                    n977 = Build Array(w1974, w1973, w1972) -> (w1963:dbl[][])
                    n978 = Index Array(array=w1961, index (row)=1) -> (element=w1971:dbl[])  [unwired: 1 in]
                    n979 = Index Array(array=w1961, index (row)=4) -> (element=w1970:dbl[])  [unwired: 1 in]
                    n980 = Index Array(array=w1961, index (row)=7) -> (element=w1969:dbl[])  [unwired: 1 in]
                    n981 = Build Array(w1971, w1970, w1969) -> (w1964:dbl[][])
                    n982 = Index Array(array=w1961, index (row)=2) -> (element=w1968:dbl[])  [unwired: 1 in]
                    n983 = Index Array(array=w1961, index (row)=5) -> (element=w1967:dbl[])  [unwired: 1 in]
                    n984 = Index Array(array=w1961, index (row)=8) -> (element=w1966:dbl[])  [unwired: 1 in]
                    n985 = Build Array(w1968, w1967, w1966) -> (w1965:dbl[][])
                    n986 = call "Canal Plane.vi"("Principal Planes"=w1965) -> ("Canal Planes"=w1960:dbl[][])
                    n987 = call "Canal Plane.vi"("Principal Planes"=w1964) -> ("Canal Planes"=w1955:dbl[][])
                    n988 = Index Array(array=w1960, index (row) #1=0 ("index (row)"), index (row) #2=1 ("index (row)")) -> (element #1=w1949:dbl[], element #2=w1946:dbl[])  [unwired: 2 in]
                    n989 = Index Array(array=w1955, index (row) #1=0 ("index (row)"), index (row) #2=1 ("index (row)")) -> (element #1=w1950:dbl[], element #2=w1947:dbl[])  [unwired: 2 in]
                    n990 = call "Canal Plane.vi"("Principal Planes"=w1963) -> ("Canal Planes"=w1952:dbl[][])
                    n991 = Index Array(array=w1952, index (row) #1=0 ("index (row)"), index (row) #2=1 ("index (row)")) -> (element #1=w1951:dbl[], element #2=w1948:dbl[])  [unwired: 2 in]
                    n992 = Build Array (concatenate)(w1961, w1951, w1950, w1949, w1948, w1947, w1946) -> (w1962:dbl[][])
                  }
                }
                n993 = Bundle(0.0, w1943, "Mean and STD"=w1938) -> (w1942:cluster{dbl, dbl, "Mean and STD":dbl[][]})  [unwired: 1 in]
                n994 = local write "Impulse Trace"(w1942) -> ()
              }
